vi "struct_abs_mix_x_pT.vi"(0 "Reference working pair (Input)":i64, 5 "Pressure in Pa (Input)":dbl, 7 "Temperature in K (Input)":dbl, 11 "Error (Input)":errorcluster) -> (4 "Mole fraction of first component liquid phase in mol/mol (Output)":dbl, 6 "Mole fraction of first component (Output)":dbl, 8 "Mole fraction of second component (Output)":dbl, 15 "Error (Output)":errorcluster)   [LabVIEW 2017]
doc: "abs_mix_x_pT:\n * -------------\n *\n * Calculates equilibrium liquid mole fraction of first component in mol/mol\n * depending on pressure in Pa and temperature T_K in K.\n *\n * Parameters:\n * -----------\n * double p_Pa:\n * Equilibrium pressure p_Pa in Pa.\n * double T_K:\n * Equilibrium temperature in K.\n * struct *WorkingPair:\n * Pointer of WorkingPair-struct.\n *\n * Returns:\n * --------\n * double:\n * Equilibrium mole fraction in of first component liquid phase in mol/mol.\n * double *ret_y_1_molmol:\n * Equilibrium mole fraction of first component.\n * double *ret_y_2_molmol:\n * Equilibrium mole fraction of second component.\n *\n * Remarks:\n * --------\n * This function is only valid for isotherm models based on mixing rules.\n *\n * History: \n * --------\n * 07/14/2021, by Jannik Driesel (supervised by Mirko Engelpracht):\n * First implementation."
uses:
  data/win32bit/libsorpPropLib.dll
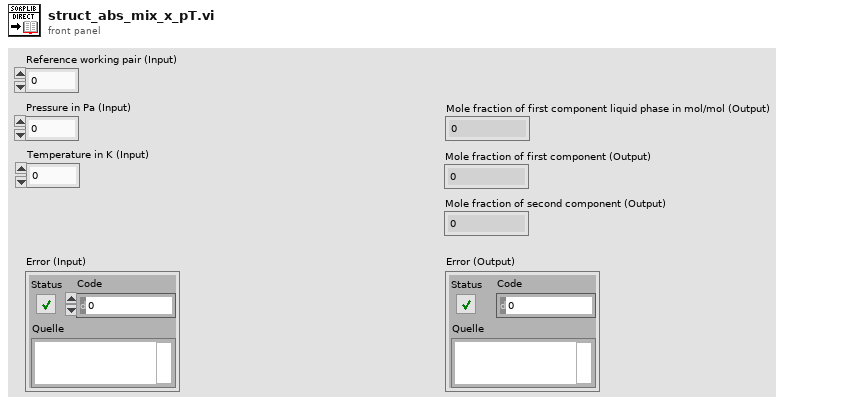
[diagram p1: front panel]
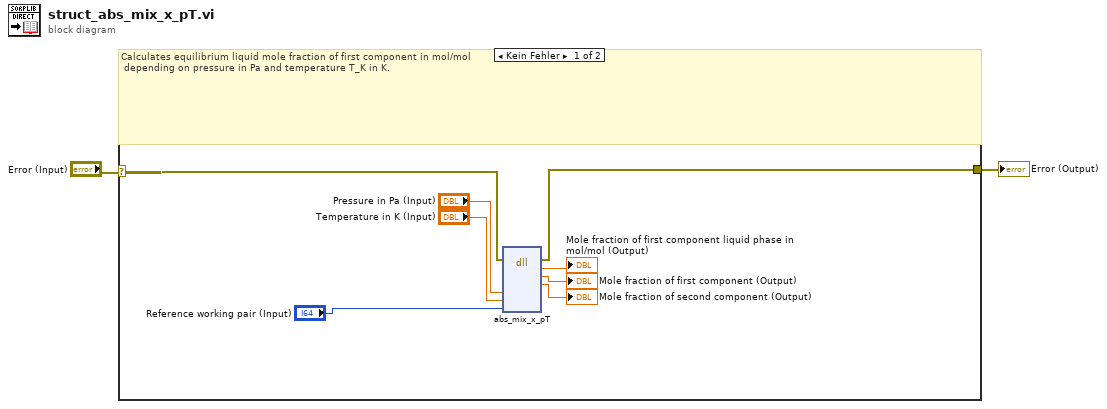
[diagram p0: block diagram]
diagram:
  n1 = case shown="Kein Fehler" "Error (Input)" {
    selector: "Error (Input)" -> [w10 w11]
    tunnel: [w9 w11] -> w2
    frame No Error {
      # "Calculates equilibrium liquid mole fraction of first component in mol/mol\n depending on pressure in Pa and temperature T_K in K."
      n2 = dll-call lib="D:/Driesel/SorpLibLocal/LabVIEW_wrapper/data/win32bit/libsorpPropLib.dll" fn="abs_mix_x_pT"(error in=w10, "p_Pa"="Pressure in Pa (Input)", "T_K"="Temperature in K (Input)", "workingPair"="Reference working pair (Input)") -> (error out=w9:errorcluster, "x_molmol"=→"Mole fraction of first component liquid phase in mol/mol (Output)":dbl, "ret_y_1_molmol"=→"Mole fraction of first component (Output)":dbl, "ret_y_2_molmol"=→"Mole fraction of second component (Output)":dbl)  [unwired: 7 in, 1 out]
    }
    frame Error {
      # "Error - No calculations"
    }
  }
  "Error (Output)" <- w2
